vi "Chop Integration Bins (VI).vi"(4 "tolerance":dbl=1e-10, 6 "data":variant, 7 "f(x)":refnum<vi>, 8 "error in (no error)":errorcluster, 10 "Chop In":bool[](array[boolean]), 11 "Bins In":cluster{"lower limit":dbl, "upper limit":dbl}[](array[cluster])) -> (0 "error out":errorcluster, 2 "Chop Out":bool[](array[boolean]), 3 "Bins Out":cluster{"lower limit":dbl, "upper limit":dbl}[](array[cluster]))   [LabVIEW 2014, in "NI_AALPro.lvlib"]
uses:
  NI_AALPro.lvlib
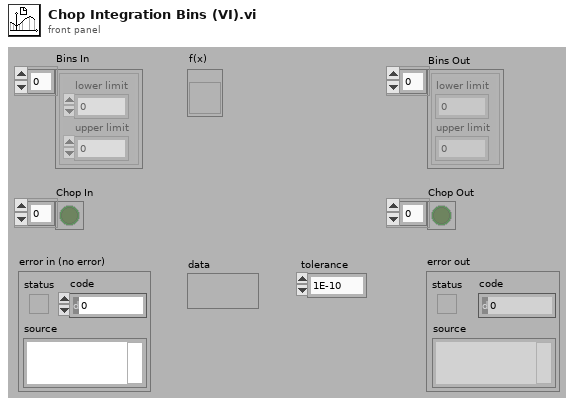
[diagram p1: front panel]
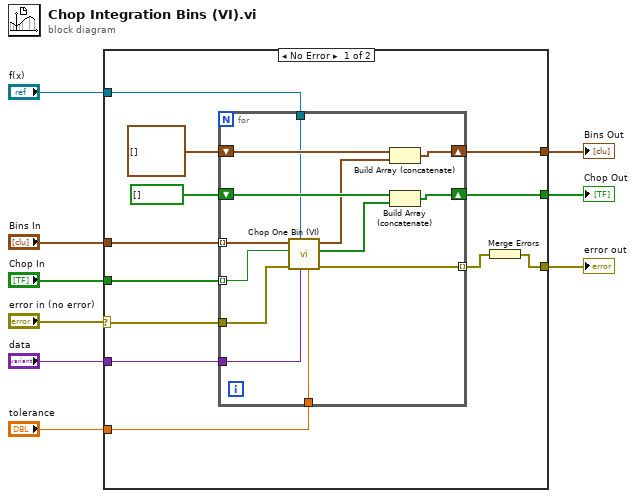
[diagram p0: block diagram]
diagram:
  n1 = case shown="No Error" "error in (no error)" {
    selector: "error in (no error)" -> [w14 w35]
    tunnel: "Bins In" -> [w21 _]
    tunnel: [w19 _] -> w8
    tunnel: "Chop In" -> [w17 _]
    tunnel: [w16 _] -> w6
    tunnel: [w11 w35] -> w5
    tunnel: "tolerance" -> [w15 _]
    tunnel: "f(x)" -> [w13 _]
    tunnel: "data" -> [w12 _]
    frame No Error {
      n2 = for {
        tunnel: w21 -> [w30] mode=indexing
        shift-right: [w32] -> w19
        shift-left: cluster{dbl, dbl}[] [] -> [w33]
        shift-right: [w34] -> w16
        shift-left: bool[] [] -> [w31]
        tunnel: w17 -> [w29] mode=indexing
        tunnel: [w26] -> w10 mode=indexing
        tunnel: w15 -> [w27]
        tunnel: w14 -> [w28]
        tunnel: w13 -> [w23]
        tunnel: w12 -> [w22]
        n3 = call "Chop One Bin (VI).vi"("tolerance"=w27, "data"=w22, "f(x)"=w23, "error in (no error)"=w28, "chop?"=w29, "bin"=w30) -> ("error out"=w26:errorcluster, "Chop Out"=w25:bool[], "Bins Out"=w24:cluster{"lower limit":dbl, "upper limit":dbl}[])  [unwired: 3 in]
        n4 = Build Array (concatenate)(w33, w24) -> (w32:cluster{"lower limit":dbl, "upper limit":dbl}[])
        n5 = Build Array (concatenate)(w31, w25) -> (w34:bool[])
      }
      n6 = Merge Errors(w10) -> (w11:errorcluster)
    }
    frame Error {
    }
  }
  "Bins Out" <- w8
  "Chop Out" <- w6
  "error out" <- w5
